vi "Arduino Parse Query Response.vi"(10 "Status":T1[](array[typedef]), 11 "input string":string) -> (2 "Status out":T1[](array[typedef]))   [LabVIEW 2021, in "FW Arduino Control.lvclass"]
uses:
  FW Arduino Control.lvclass
  Filter Wheel Object/Filter Wheel Motor Status.ctl
  <vilib>/regexp/Match Regular Expression.xnode
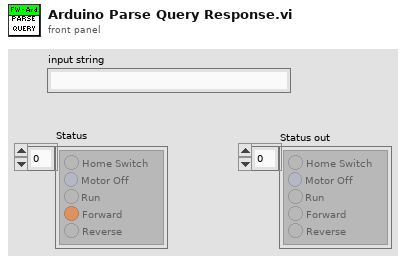
[diagram p1: front panel]
types:
  T1 = typedef "Filter Wheel Motor Status.ctl" = cluster{"Home Switch":bool, "Motor Off":bool, "Run":bool, "Forward":bool, "Reverse":bool}
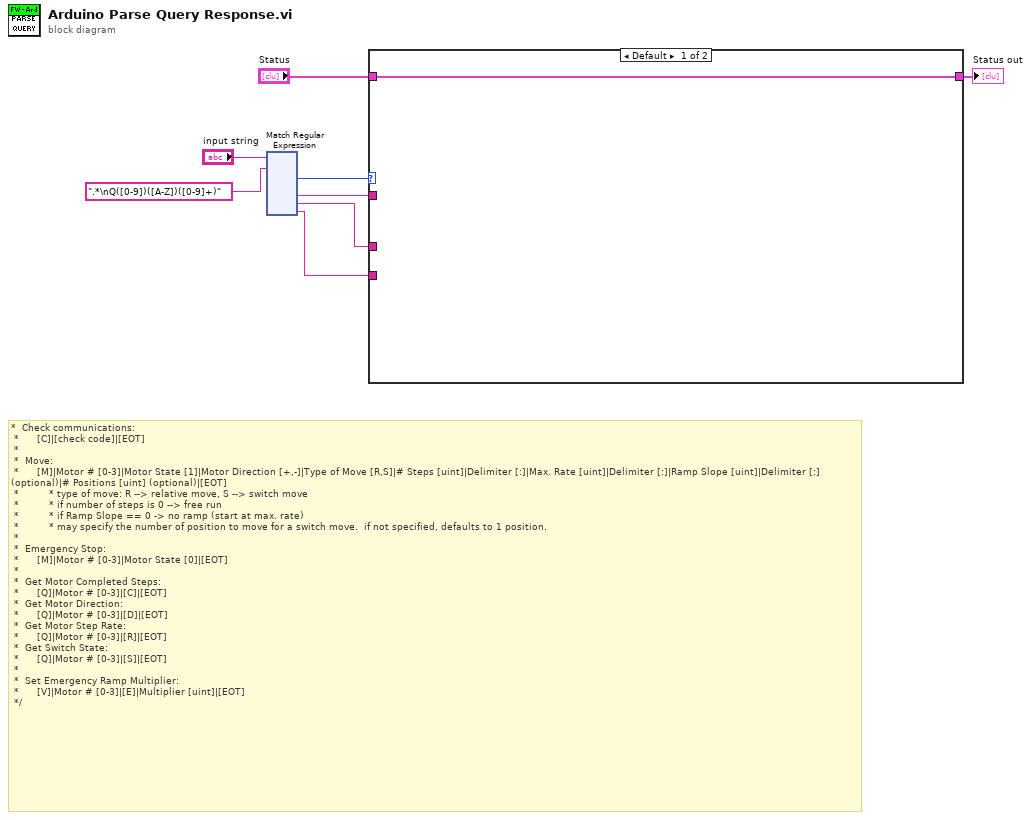
[diagram p0: block diagram]
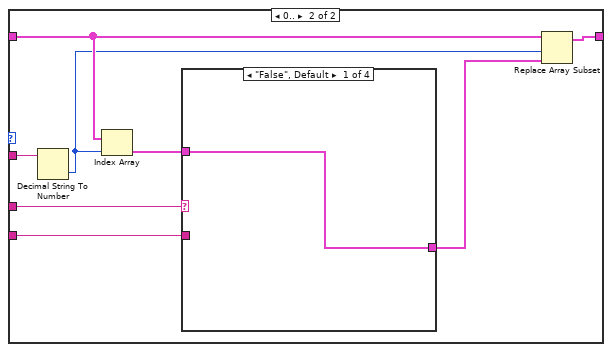
[diagram p2: hidden frame]
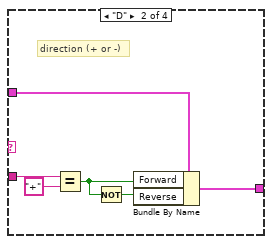
[diagram p3: hidden frame]
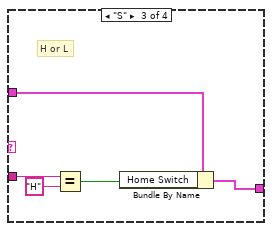
[diagram p4: hidden frame]
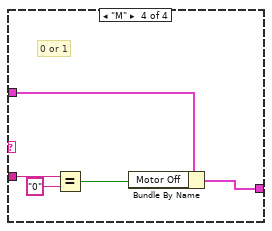
[diagram p5: hidden frame]
diagram:
  # "*  Check communications:\n *      [C]|[check code]|[EOT]\n *\n *  Move:\n *      [M]|Motor # [0-3]|Motor State [1]|Motor Direction [+,-]|Type of Move [R,S]|# Steps [uint]|Delimiter [:]|Max. Rate [uint]|Delimiter [:]|Ramp Slope [uint]|Delimiter [:] (optional)|# Positions [uint] (optional)|[EOT]\n *          * type of move: R --> relative move, S --> switch move\n *          * if number of steps is 0 --> free run\n *          * if Ramp Slope == 0 -> no ramp (start at max. rate)\n *          * may specify the number of position to move for a switch move.  if not specified, defaults to 1 position.\n *\n *  Emergency Stop:\n *      [M]|Motor # [0-3]|Motor State [0]|[EOT]\n *\n *  Get Motor Completed Steps:\n *      [Q]|Motor # [0-3]|[C]|[EOT]\n *  Get Motor Direction:\n *      [Q]|Motor # [0-3]|[D]|[EOT]\n *  Get Motor Step Rate:\n *      [Q]|Motor # [0-3]|[R]|[EOT]\n *  Get Switch State:\n *      [Q]|Motor # [0-3]|[S]|[EOT]\n *\n *  Set Emergency Ramp Multiplier:\n *      [V]|Motor # [0-3]|[E]|Multiplier [uint]|[EOT]\n */"
  n1 = xnode "Match Regular Expression"("input string"="input string", "regular expression"=".*\nQ([0-9])([A-Z])([0-9]+)") -> ("offset past match"=w8:i32, "submatch 1"=w5:string, "submatch 2"=w4:string, "submatch 3"=w3:string)  [unwired: 4 in, 4 out]
  n2 = case shown="Default" w8 {
    tunnel: w5 -> [_ w17]
    tunnel: w4 -> [_ w16]
    tunnel: w3 -> [_ w15]
    tunnel: "Status" -> [w9 w13]
    tunnel: [w9 w10] -> w1
    frame Default {
    }
    frame 0.. {
      n3 = Decimal String To Number(string=w17) -> (number=w12:i32)  [unwired: 2 in, 1 out]
      n4 = Index Array(array=w13, index=w12) -> (element=w14:T1)
      n5 = case shown="\"False\", Default" w16 {
        tunnel: w15 -> [_ w24 w29 w34]
        tunnel: w14 -> [w18 w22 w27 w32]
        tunnel: [w18 w19 w25 w30] -> w11
        frame "False", Default {
        }
        frame "D" {
          # "direction (+ or -)"
          n6 = Equal?(x=w24, y="+") -> (x = y?=w20:bool)
          n7 = Not(x=w20) -> (.not. x?=w21:bool)
          n8 = Bundle By Name(cluster=w22, "Forward"=w20, "Reverse"=w21) -> (w19:T1)
        }
        frame "S" {
          # "H or L"
          n9 = Equal?(x=w29, y="H") -> (x = y?=w26:bool)
          n10 = Bundle By Name(cluster=w27, "Home Switch"=w26) -> (w25:T1)
        }
        frame "M" {
          # "0 or 1"
          n11 = Equal?(x=w34, y="0") -> (x = y?=w31:bool)
          n12 = Bundle By Name(cluster=w32, "Motor Off"=w31) -> (w30:T1)
        }
      }
      n13 = Replace Array Subset(array=w13, new element=w11, index=w12) -> (w10:T1[])
    }
  }
  "Status out" <- w1
